vi "CreatCom1.vi"(8 "error in (no error)":errorcluster, 9 "Serial Settings":T1={"baud rate"=57600, "data bits"=8, "parity"=enum."None", "stop bits"=10, "flow control"=0} {"flow control" items=["None"=0, "XON/XOFF"=1, "RTS/CTS"=2, "DTR/DSR"=4]; "stop bits" items=["1.0"=10, "1.5"=15, "2.0"=20]; "data bits" min=5 max=8 step=1; "baud rate" items=["75"=75, "110"=110, "134"=134, "150"=150, "300"=300, "600"=600, "1200"=1200, "1800"=1800, "2400"=2400, "4800"=4800, "7200"=7200, "9600"=9600, "14400"=14400, "19200"=19200, "28800"=28800, "38400"=38400, "56000"=56000, "57600"=57600, "115200"=115200, "128000"=128000, "230400"=230400]}, 11 "COM":string) -> (0 "error out":errorcluster, 3 "COM1":refnum<visa-resource-name>)   [LabVIEW 2014]
uses:
  <vilib>/Instr/_visa.llb/VISA Configure Serial Port (Instr).vi
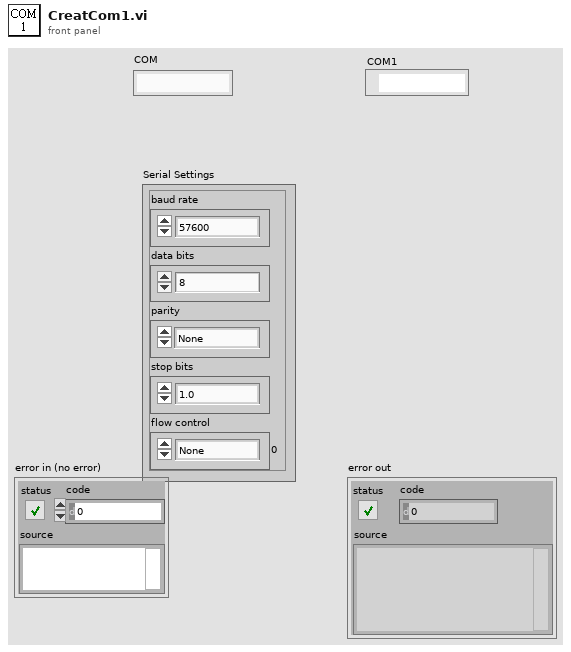
[diagram p1: front panel]
types:
  T1 = cluster{"baud rate":u32, "data bits":u16, "parity":enum16{"None", "Odd", "Even", "Mark", "Space"}, "stop bits":u16, "flow control":u16}
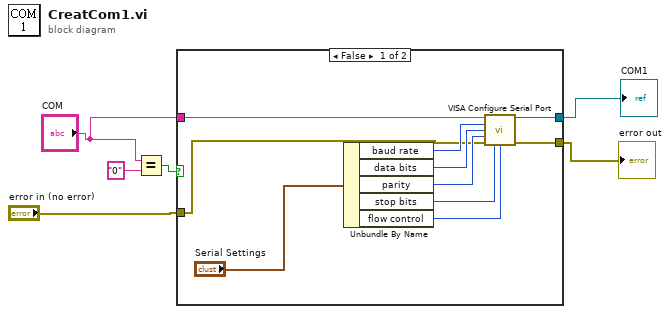
[diagram p0: block diagram]
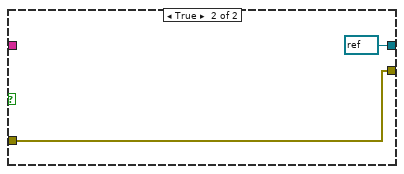
[diagram p2: hidden frame]
diagram:
  n1 = Equal?(x="COM", y="0") -> (x = y?=w3:bool)
  n2 = case shown="False" w3 {
    tunnel: "COM" -> [w10 _]
    tunnel: [w9 w18] -> w5
    tunnel: "error in (no error)" -> [w8 w18]
    tunnel: [w7 refnum<visa-resource-name> refnum ("VISA resource name out")] -> w1
    frame False {
      n3 = Unbundle By Name("Serial Settings") -> ("baud rate"=w12:u32, "data bits"=w11:u16, "parity"=w14:enum16{"None", "Odd", "Even", "Mark", "Space"}, "stop bits"=w15:u16, "flow control"=w16:u16)
      n4 = call-poly "VISA Configure Serial Port"("VISA resource name"=w10, "baud rate (9600)"=w12, "data bits (8)"=w11, "parity (0:none)"=w14, "error in (no error)"=w8, "stop bits (10: 1 bit)"=w15, "flow control (0:none)"=w16) -> ("VISA resource name out"=w7:refnum<visa-resource-name>, "error out"=w9:errorcluster)  [unwired: 2 in, 5 out]
    }
    frame True {
    }
  }
  "error out" <- w5
  "COM1" <- w1
